vi "Control_BSA_setup.vi"(0 "setup":T1, 7 "BSA number":string) -> ()   [LabVIEW 2010]
uses:
  Controls/Setup.ctl
  Globals/Meas_global.vi
  Globals/LDA_meas_global_2.vi
  Globals/LDA_meas_global_1.vi
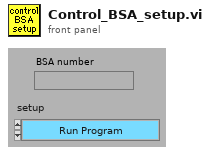
[diagram p1: front panel]
types:
  T1 = typedef "Setup.ctl" = enum16{"Run Program", "Show Setup", "Save Current Setup", "Setup Front Panel"}
  T2 = enum16{"Velocity", "Transit time", "Arrival time"}
  T3 = typedef "BSA_info_Cluster.ctl" = cluster{"GPIB Address":string, "No of Check Bytes":i32, "Extra Info":string, "COLOUR":u32, "Wavelength (nm)":dbl}
  T4 = cluster{"Output data format":enum16{"Velocity, transit time, arrival time", "Velocity, arrival time", "Velocity, transit time", "Velocity"}, "Non-validated signals":enum16{"Accept", "Reject"}}
  T5 = cluster{"High voltage":i16, "Signal gain (dB)":i16}
  T6 = enum16{"6.4", "3.2", "1.6", "0.8", "0.4", "0.2", "0.1", "0.05"}
  T7 = cluster{"Centre Velocity":u16, "Velocity span":u16, "Units":enum16{"Hz", "m/s"}, "Frequency shift":enum16{"Disabled", "Enabled"}}
  T8 = cluster{"Arrival time clock":enum16{"External", "Internal"}, "Clock source":enum16{"Slave", "Master", "Private"}, "Coincidence":enum16{"Slave", "Master", "Private"}}
  T9 = cluster{"Dead time (s)":dbl, "Duty cycle (%)":dbl, "Data collection mode":enum16{"Burst", "Contiuous", "Dead time", "External"}}
  T10 = cluster{"Burst criterion":enum16{"Envelope", "Pedestal", "Env and ped"}, "Oversize reject level":enum16{"1 (disabled)", "2", "3", "4", "5", "6", "7", "8", "9"}, "Pedestal attenuation":enum16{"0", "6", "12", "18"}, "Record length":enum16{"8", "16", "32", "64"}, "Quality factor":i16}
  T11 = cluster{"Centre frequency":u16, "Bandwidth":u16, "Units":enum16{"Hz", "m/s"}, "Frequency shift":enum16{"Disabled", "Enabled"}}
  T12 = enum16{"Velocity, transit time, arrival time", "Velocity, arrival time", "Velocity, transit time", "Velocity"}
  T13 = enum16{"Velocity", "Transit time", "Arrival time"}[]
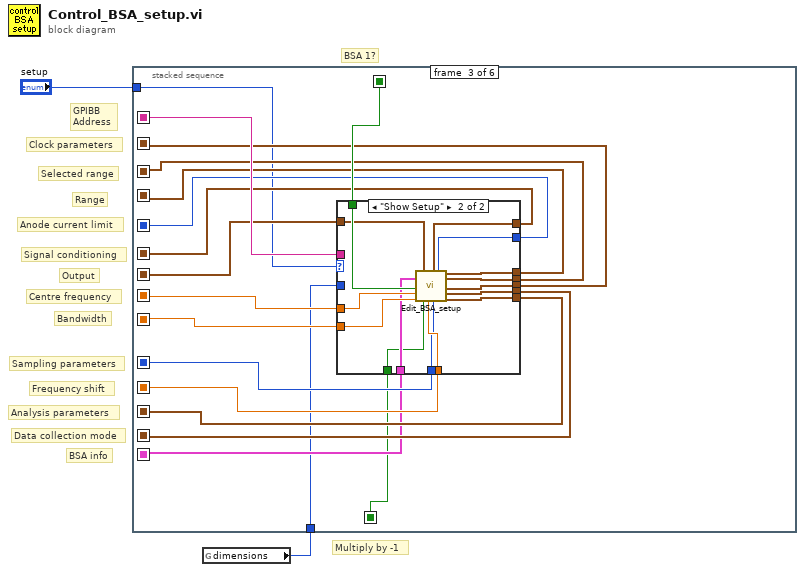
[diagram p0: block diagram]
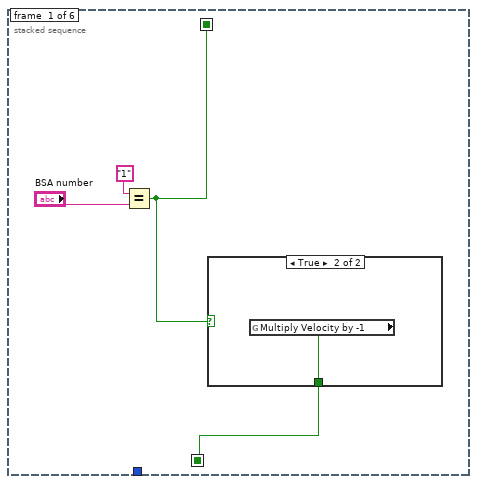
[diagram p2: hidden frame]
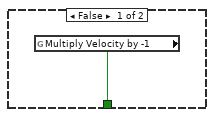
[diagram p3: hidden frame]
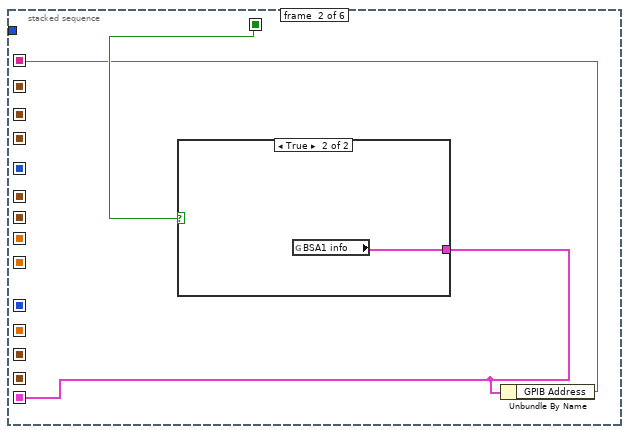
[diagram p4: hidden frame]
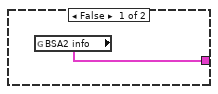
[diagram p5: hidden frame]
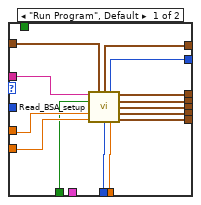
[diagram p6: hidden frame]
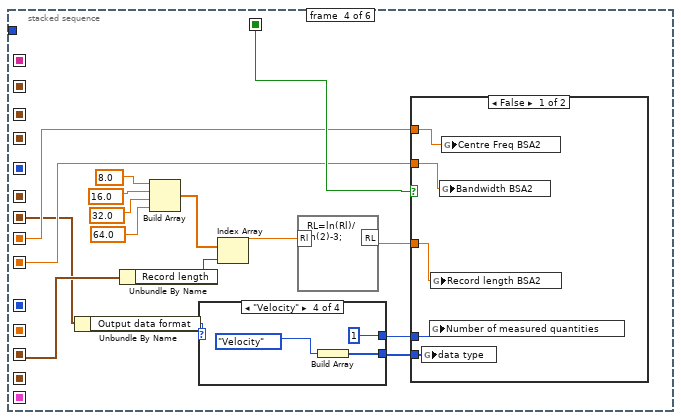
[diagram p7: hidden frame]
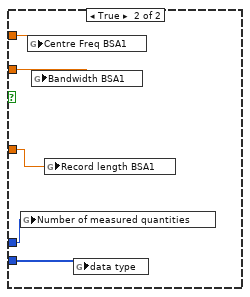
[diagram p8: hidden frame]
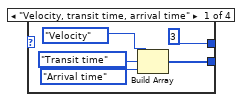
[diagram p9: hidden frame]
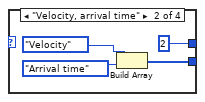
[diagram p10: hidden frame]
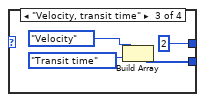
[diagram p11: hidden frame]
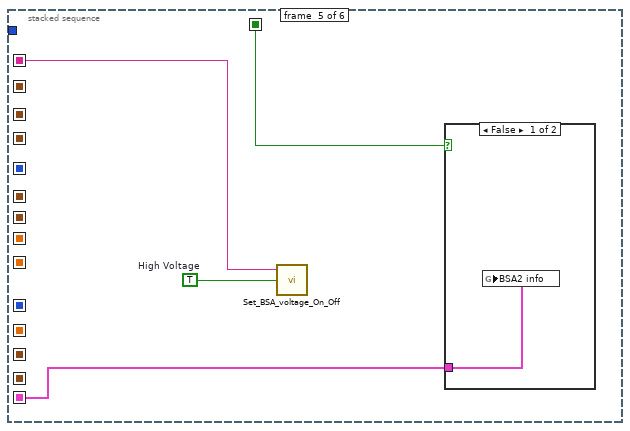
[diagram p12: hidden frame]
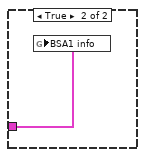
[diagram p13: hidden frame]
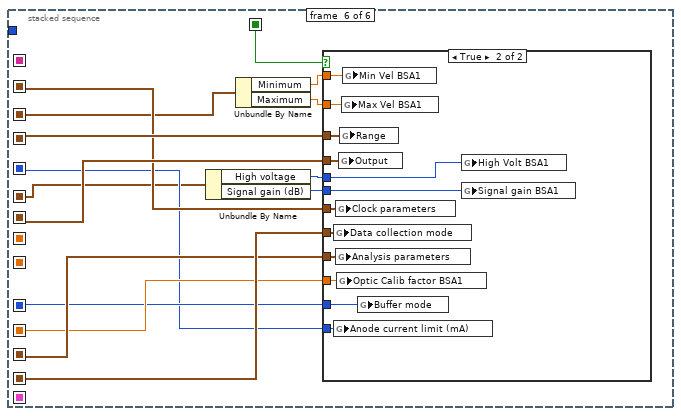
[diagram p14: hidden frame]
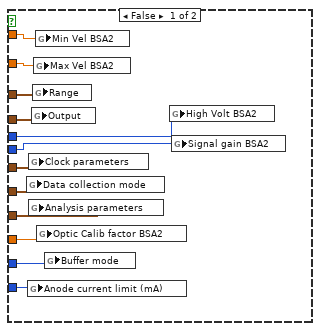
[diagram p15: hidden frame]
diagram:
  # "Multiply by -1"
  # "Bandwidth"
  # "Centre frequency"
  # "Anode current limit"
  # "Selected range"
  # "Range"
  # "Signal conditioning"
  # "Analysis parameters"
  # "Data collection mode"
  # "Frequency shift"
  # "Output"
  # "Clock parameters"
  # "Sampling parameters"
  # "BSA 1?"
  # "BSA info"
  # "GPIBB\nAddress"
  n1 = global read "Meas_global.vi" "dimensions"() -> (w1:enum16{"1D", "2D"})
  n2 = stacked-sequence {
    seq-local: [_ _ w29 _ _ _] -> [_ _ _ _ _ w119]
    seq-local: [_ w9 _ _ _ _] -> [_ _ w31 _ w103 _]
    seq-local: [_ w10 _ _ _ _] -> [_ _ w17 _ w106 _]
    seq-local: [w4 _ _ _ _ _] -> [_ w11 w30 w71 w105 w123]
    seq-local: [_ _ w22 _ _ _] -> [_ _ _ _ _ w111]
    seq-local: [_ _ w23 _ _ _] -> [_ _ _ _ _ w122]
    seq-local: [_ _ w24 _ _ _] -> [_ _ _ _ _ w115]
    seq-local: [_ _ w25 _ _ _] -> [_ _ _ _ _ w114]
    seq-local: [_ _ w26 _ _ _] -> [_ _ _ _ _ w116]
    seq-local: [_ _ w27 _ _ _] -> [_ _ _ _ _ w117]
    seq-local: [_ _ w28 _ _ _] -> [_ _ _ w68 _ w118]
    seq-local: [_ _ w21 _ _ _] -> [_ _ _ _ _ w120]
    seq-local: [_ _ w20 _ _ _] -> [_ _ _ w61 _ w121]
    seq-local: [_ _ w19 _ _ _] -> [_ _ _ w70 _ _]
    seq-local: [_ _ w18 _ _ _] -> [_ _ _ w69 _ _]
    seq-local: [w3 _ _ _ _ _] -> [_ _ w14 _ _ _]
    tunnel: w1 -> [_ _ w16 _ _ _]
    tunnel: "setup" -> [_ _ w15 _ _ _]
    frame #0 {
      n3 = Equal?(x="1", y="BSA number") -> (x = y?=w4:bool)
      n4 = case shown="True" w4 {
        tunnel: [w7 w8] -> w3
        frame False {
          n5 = global read "LDA_meas_global_2.vi" "Multiply Velocity by -1"() -> (w7:bool)
        }
        frame True {
          n6 = global read "LDA_meas_global_1.vi" "Multiply Velocity by -1"() -> (w8:bool)
        }
      }
    }
    frame #1 {
      n7 = case shown="True" w11 {
        tunnel: [w12 w13] -> w10
        frame False {
          n8 = global read "LDA_meas_global_2.vi" "BSA2 info"() -> (w12:T3)
        }
        frame True {
          n9 = global read "LDA_meas_global_1.vi" "BSA1 info"() -> (w13:T3)
        }
      }
      n10 = Unbundle By Name(w10) -> ("GPIB Address"=w9:string)
    }
    frame #2 {
      n11 = case shown="\"Show Setup\"" w15 {
        tunnel: w31 -> [w45 _]
        tunnel: w30 -> [_ w60]
        tunnel: [w44 w59] -> w23
        tunnel: [w43 w58] -> w22
        tunnel: [w42 w57] -> w21
        tunnel: [w41 w56] -> w29
        tunnel: [w40 w55] -> w28
        tunnel: [w39 w54] -> w27
        tunnel: [w38 w53] -> w26
        tunnel: [w37 w52] -> w25
        tunnel: [w36 w51] -> w24
        tunnel: [w35 w50] -> w20
        tunnel: [w34 w49] -> w19
        tunnel: [w33 w48] -> w18
        tunnel: w17 -> [_ w47]
        tunnel: w16 -> [_ _]
        tunnel: w14 -> [w32 w46]
        frame "Run Program", Default {
          n12 = call "Read_BSA_setup.vi"("GPIB Address"=w45, "Multiply Velocity by -1"=w32) -> ("Output"=w35:T4, "Signal conditioning"=w37:T5, "Anode current limit (mA)"=w36:T6, "Range"=w44:T7, "Selected range"=w43:cluster{"Minimum":dbl, "Maximum":dbl}, "Clock parameters"=w42:T8, "Centre frequency"=w34:dbl, "Data collection mode"=w41:T9, "Bandwidth"=w33:dbl, "Buffer mode"=w38:enum16{"One shot", "Ring", "FIFO"}, "Calibration factor"=w39:dbl, "Analysis parameters"=w40:T10)  [unwired: 1 in, 1 out]
        }
        frame "Show Setup" {
          n13 = call "Edit_BSA_setup.vi"("BSA info"=w47, "BSA 1?"=w60, "Multiply Velocity by -1"=w46) -> ("Centre frequency"=w49:dbl, "Bandwidth"=w48:dbl, "Output"=w50:T4, "Calibration factor"=w54:dbl, "Signal conditioning (out)"=w52:T5, "Buffer mode out"=w53:enum16{"One shot", "Ring", "FIFO"}, "Anode current limit (mA)"=w51:T6, "Range (out)"=w59:T11, "Selected range"=w58:cluster{"Minimum":dbl, "Maximum":dbl}, "Clock parameters (out)"=w57:T8, "Data collection mode (out)"=w56:T9, "Analysis parameters (out)"=w55:T10)  [unwired: 1 in, 4 out]
        }
      }
    }
    frame #3 {
      n14 = Unbundle By Name(w61) -> ("Output data format"=w75:T12)
      n15 = Unbundle By Name(w68) -> ("Record length"=w76:enum16{"8", "16", "32", "64"})
      n16 = Build Array(8.0, 16.0, 32.0, 64.0) -> (w63:dbl[])
      n17 = case shown="\"Velocity\"" w75 {
        tunnel: [3 2 2 1] -> w73
        tunnel: [w90 w94 w97 w101] -> w74
        frame "Velocity, transit time, arrival time" {
          n18 = Build Array(T2."Velocity", T2."Transit time", T2."Arrival time") -> (w90:T13)
        }
        frame "Velocity, arrival time" {
          n19 = Build Array(T2."Velocity", T2."Arrival time") -> (w94:T13)
        }
        frame "Velocity, transit time" {
          n20 = Build Array(T2."Velocity", T2."Transit time") -> (w97:T13)
        }
        frame "Velocity" {
          n21 = Build Array(T2."Velocity") -> (w101:T13)
        }
      }
      n22 = Index Array(array=w63, index=w76) -> (element=w62:dbl)
      n23 = formula code="RL=ln(Rl)/ln(2)-3;"("Rl"=w62) -> ("RL"=w72:dbl)
      n24 = case shown="False" w71 {
        tunnel: w70 -> [w77 w86]
        tunnel: w74 -> [w81 w85]
        tunnel: w73 -> [w80 w84]
        tunnel: w72 -> [w79 w83]
        tunnel: w69 -> [w78 w82]
        frame False {
          n25 = global write "LDA_meas_global_2.vi" "data type"(w81) -> ()
          n26 = global write "LDA_meas_global_2.vi" "Number of measured quantities"(w80) -> ()
          n27 = global write "LDA_meas_global_2.vi" "Record length BSA2"(w79) -> ()
          n28 = global write "LDA_meas_global_2.vi" "Bandwidth BSA2"(w78) -> ()
          n29 = global write "LDA_meas_global_2.vi" "Centre Freq BSA2"(w77) -> ()
        }
        frame True {
          n30 = global write "LDA_meas_global_1.vi" "Number of measured quantities"(w84) -> ()
          n31 = global write "LDA_meas_global_1.vi" "Centre Freq BSA1"(w86) -> ()
          n32 = global write "LDA_meas_global_1.vi" "Bandwidth BSA1"(w82) -> ()
          n33 = global write "LDA_meas_global_1.vi" "Record length BSA1"(w83) -> ()
          n34 = global write "LDA_meas_global_1.vi" "data type"(w85) -> ()
        }
      }
    }
    frame #4 {
      w104 = TRUE  # High Voltage
      n35 = call "Set_BSA_voltage_On_Off.vi"("GPIB address"=w103, "High Voltage"=w104) -> ()  [unwired: 1 in, 5 out]
      n36 = case shown="False" w105 {
        tunnel: w106 -> [w107 w108]
        frame False {
          n37 = global write "LDA_meas_global_2.vi" "BSA2 info"(w107) -> ()
        }
        frame True {
          n38 = global write "LDA_meas_global_1.vi" "BSA1 info"(w108) -> ()
        }
      }
    }
    frame #5 {
      n39 = Unbundle By Name(w114) -> ("High voltage"=w113:i16, "Signal gain (dB)"=w112:i16)
      n40 = Unbundle By Name(w111) -> ("Minimum"=w110:dbl, "Maximum"=w109:dbl)
      n41 = case shown="True" w123 {
        tunnel: w122 -> [w135 w147]
        tunnel: w121 -> [w134 w146]
        tunnel: w120 -> [w133 w145]
        tunnel: w119 -> [w132 w144]
        tunnel: w118 -> [w131 w143]
        tunnel: w117 -> [w130 w142]
        tunnel: w116 -> [w129 w141]
        tunnel: w115 -> [w128 w140]
        tunnel: w113 -> [w127 w139]
        tunnel: w112 -> [w126 w138]
        tunnel: w110 -> [w125 w137]
        tunnel: w109 -> [w124 w136]
        frame False {
          n42 = global write "LDA_meas_global_2.vi" "Data collection mode"(w132) -> ()
          n43 = global write "LDA_meas_global_2.vi" "Anode current limit (mA)"(w128) -> ()
          n44 = global write "LDA_meas_global_2.vi" "Clock parameters"(w133) -> ()
          n45 = global write "LDA_meas_global_2.vi" "Analysis parameters"(w131) -> ()
          n46 = global write "LDA_meas_global_2.vi" "Output"(w134) -> ()
          n47 = global write "LDA_meas_global_2.vi" "Range"(w135) -> ()
          n48 = global write "LDA_meas_global_2.vi" "Max Vel BSA2"(w124) -> ()
          n49 = global write "LDA_meas_global_2.vi" "Min Vel BSA2"(w125) -> ()
          n50 = global write "LDA_meas_global_2.vi" "Optic Calib factor BSA2"(w130) -> ()
          n51 = global write "LDA_meas_global_2.vi" "Buffer mode"(w129) -> ()
          n52 = global write "LDA_meas_global_2.vi" "High Volt BSA2"(w127) -> ()
          n53 = global write "LDA_meas_global_2.vi" "Signal gain BSA2"(w126) -> ()
        }
        frame True {
          n54 = global write "LDA_meas_global_1.vi" "Data collection mode"(w144) -> ()
          n55 = global write "LDA_meas_global_1.vi" "Anode current limit (mA)"(w140) -> ()
          n56 = global write "LDA_meas_global_1.vi" "Clock parameters"(w145) -> ()
          n57 = global write "LDA_meas_global_1.vi" "Analysis parameters"(w143) -> ()
          n58 = global write "LDA_meas_global_1.vi" "Optic Calib factor BSA1"(w142) -> ()
          n59 = global write "LDA_meas_global_1.vi" "Output"(w146) -> ()
          n60 = global write "LDA_meas_global_1.vi" "Range"(w147) -> ()
          n61 = global write "LDA_meas_global_1.vi" "Max Vel BSA1"(w136) -> ()
          n62 = global write "LDA_meas_global_1.vi" "Min Vel BSA1"(w137) -> ()
          n63 = global write "LDA_meas_global_1.vi" "Buffer mode"(w141) -> ()
          n64 = global write "LDA_meas_global_1.vi" "High Volt BSA1"(w139) -> ()
          n65 = global write "LDA_meas_global_1.vi" "Signal gain BSA1"(w138) -> ()
        }
      }
    }
  }
